vi "pid array element to PID Loop Object.vi"(8 "error in (no error)":errorcluster, 11 "PID Element in":T1) -> (0 "error out":errorcluster, 3 "PID Loop out":refnum<class "PID Loop.lvclass">)   [LabVIEW 2015, in "PID Loop.lvclass"]
uses:
  PID Loop.lvclass
  editor node/PID array element.ctl
  PID Loop/PID Parameters.ctl
  PID Loop/PID Gains.ctl
  PID Loop/PID Range.ctl
  PID Module configuration.lvclass
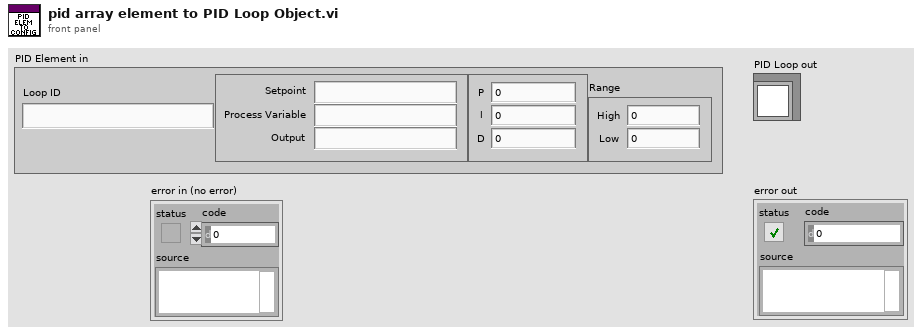
[diagram p1: front panel]
types:
  T1 = typedef "PID Module configuration.lvclass/PID array element.ctl" = cluster{"Loop ID":string, "Tags":cluster{"Setpoint":string, "Process Variable":string, "Output":string}, "Gains":cluster{"P":dbl, "I":dbl, "D":dbl}, "Range":cluster{"High":dbl, "Low":dbl}}
  T2 = typedef "PID Loop.lvclass/PID Range.ctl" = cluster{"output high":dbl, "output low":dbl}
  T3 = typedef "PID Loop.lvclass/PID Gains.ctl" = cluster{"proportional gain (Kc)":dbl, "integral time (Ti, min)":dbl, "derivative time (Td, min)":dbl}
  T4 = typedef "PID Loop.lvclass/PID Parameters.ctl" = cluster{"Setpoint Tag":string, "Process Variable Tag":string, "Output Tag":string}
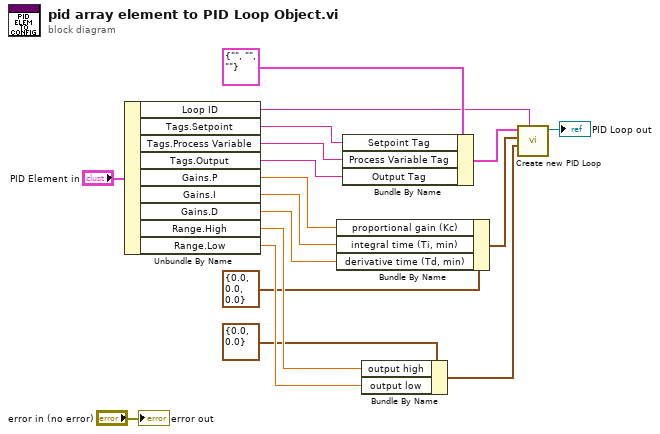
[diagram p0: block diagram]
diagram:
  n1 = Unbundle By Name("PID Element in") -> ("Loop ID"=w3:string, "Tags.Setpoint"=w7:string, "Tags.Process Variable"=w8:string, "Tags.Output"=w9:string, "Gains.P"=w11:dbl, "Gains.I"=w12:dbl, "Gains.D"=w13:dbl, "Range.High"=w16:dbl, "Range.Low"=w17:dbl)
  n2 = Bundle By Name(cluster=T3 {"proportional gain (Kc)"=0.0, "integral time (Ti, min)"=0.0, "derivative time (Td, min)"=0.0} ("PID gains"), "proportional gain (Kc)"=w11, "integral time (Ti, min)"=w12, "derivative time (Td, min)"=w13) -> (w14:T3)
  n3 = Bundle By Name(cluster=T4 {"Setpoint Tag"="", "Process Variable Tag"="", "Output Tag"=""} ("PID Parameters"), "Setpoint Tag"=w7, "Process Variable Tag"=w8, "Output Tag"=w9) -> (w6:T4)
  n4 = Bundle By Name(cluster=T2 {"output high"=0.0, "output low"=0.0} ("output range"), "output high"=w16, "output low"=w17) -> (w18:T2)
  n5 = call "Create new PID Loop.vi"("ID"=w3, "output range"=w18, "PID gains"=w14, "PID Parameters"=w6) -> ("PID Loop out"=→"PID Loop out":refnum<class "PID Loop.lvclass">)  [unwired: 6 in, 1 out]
  "error out" <- "error in (no error)"
